vi "Joystick Get.vi"(8 "reset":bool, 9 "JoystickRefDrive 2":T2={"Device"=enum."USB 1"}, 10 "JoystickRefOp":T2={"Device"=enum."USB 1"}, 11 "JoystickRefDrive":T2={"Device"=enum."USB 1"}) -> ()   [LabVIEW 2014]
uses:
  <vilib>/Rock Robotics/WPI/Joystick/WPI_JoystickDevRef.ctl
  <vilib>/Rock Robotics/WPI/Joystick/WPI_JoystickDeviceEnum.ctl
  AxisLayoutOpJoyReg.ctl
  ButtonLayoutOpJoyReg.ctl
  ButtonLayoutDriveJoyReg.ctl
  Events.vi
  <vilib>/ptbypt/NI_PtbyPt.lvlib
panel:
  in  "PID gains 2":T1={"proportional gain (Kc)"=0.030222000000000006, "integral time (Ti, min)"=0.025000000000000015, "derivative time (Td, min)"=0.0} {"derivative time (Td, min)" format="%.3f"; "integral time (Ti, min)" format="%.3f"; "proportional gain (Kc)" format="%.3f"}
  in  "PID gains":T1={"proportional gain (Kc)"=2.0, "integral time (Ti, min)"=0.1, "derivative time (Td, min)"=0.0} {"derivative time (Td, min)" format="%.3f"; "integral time (Ti, min)" format="%.3f"; "proportional gain (Kc)" format="%.3f"}
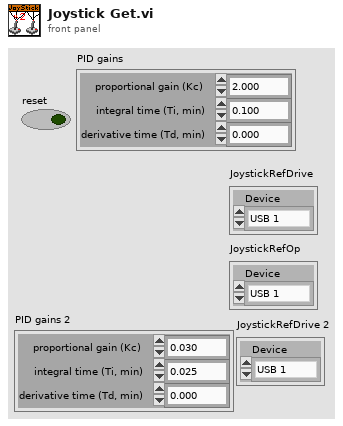
[diagram p1: front panel]
types:
  T1 = cluster{"proportional gain (Kc)":dbl, "integral time (Ti, min)":dbl, "derivative time (Td, min)":dbl}
  T2 = typedef "WPI_JoystickDevRef.ctl" = cluster{"Device":T3}
  T3 = typedef "WPI_JoystickDeviceEnum.ctl" = enum16{"USB 0", "USB 1", "USB 2", "USB 3", "USB 4", "USB 5"}
  T4 = typedef "ButtonLayoutDriveJoyReg.ctl" = cluster{"Ring light":bool, "Button 2":bool, "Button 3":bool, "Button 4":bool, "ShiftLow":bool, "ShiftHigh":bool, "Button 7":bool, "Button 8":bool, " Recalibrate":bool, "Exponential drive":bool, "Button 11":bool, "Button 12":bool}
  T5 = typedef "ButtonLayoutOpJoyReg.ctl" = cluster{"Accq Shoulder":bool, "Reload":bool, "Manuall truss servo":bool, "Button 4":bool, "Pass":bool, "Grab":bool, "Trajectory ctl":bool, "Throw":bool, "Accq Shoulder up":bool, "Button 10":bool, "Button 11":bool, "Button 12":bool}
  T6 = typedef "AxisLayoutOpJoyReg.ctl" = cluster{"axis 1":dbl, "axis 2":dbl, "axis 3":dbl, "axis 4":dbl, "axis 5":dbl, "Change Power":dbl}
  T7 = cluster{"OpJoyType":string, "DriveJoyType":string}
  T8 = cluster{"Translate":dbl, "Y-Axis (Backward Speed)":dbl, "Rotate":dbl, "Tank right side":dbl, "axis 5":dbl, "axis 6":dbl, "Use gyro":bool, "Exponential\ndrive":bool, "Ring light":bool, "PID rotation":bool, "PID Gain":dbl}
  T9 = cluster{"Button 1":bool, "Button 2":bool, "Button 3":bool, "Button 4":bool, "Button 5":bool, "Button 6":bool, "Button 7":bool, "Button 8":bool, "Button 9":bool, "Button 10":bool, "Button 11":bool, "Button 12":bool}
  T10 = cluster{"axis 1 (x)":dbl, "axis 2 (y)":dbl, "axis 3 (throttle)":dbl, "axis 4":dbl, "axis 5":dbl, "axis 6":dbl}
  T11 = typedef "WPI_SolenoidValue.ctl" = enum16{"Off", "On", "Forward", "Reverse"}
  T12 = cluster{"Ultrasonic Distance (In)":dbl, "Gyro":dbl, "TopAquisition sensor":bool, "Encoder distance":dbl, "Encoder rate":dbl, "Encoder direction":bool, "winch engaged?":T11, "Motor Values":dbl[], "Latch encoder":u32, "BottomAquistion":bool, "BottomAquistion 2":bool, "Gyro Rate":dbl}
  T13 = cluster{"axis 1":dbl, "axis 2":dbl, "axis 3":dbl, "axis 4":dbl, "axis 5":dbl, "Change Power":dbl}
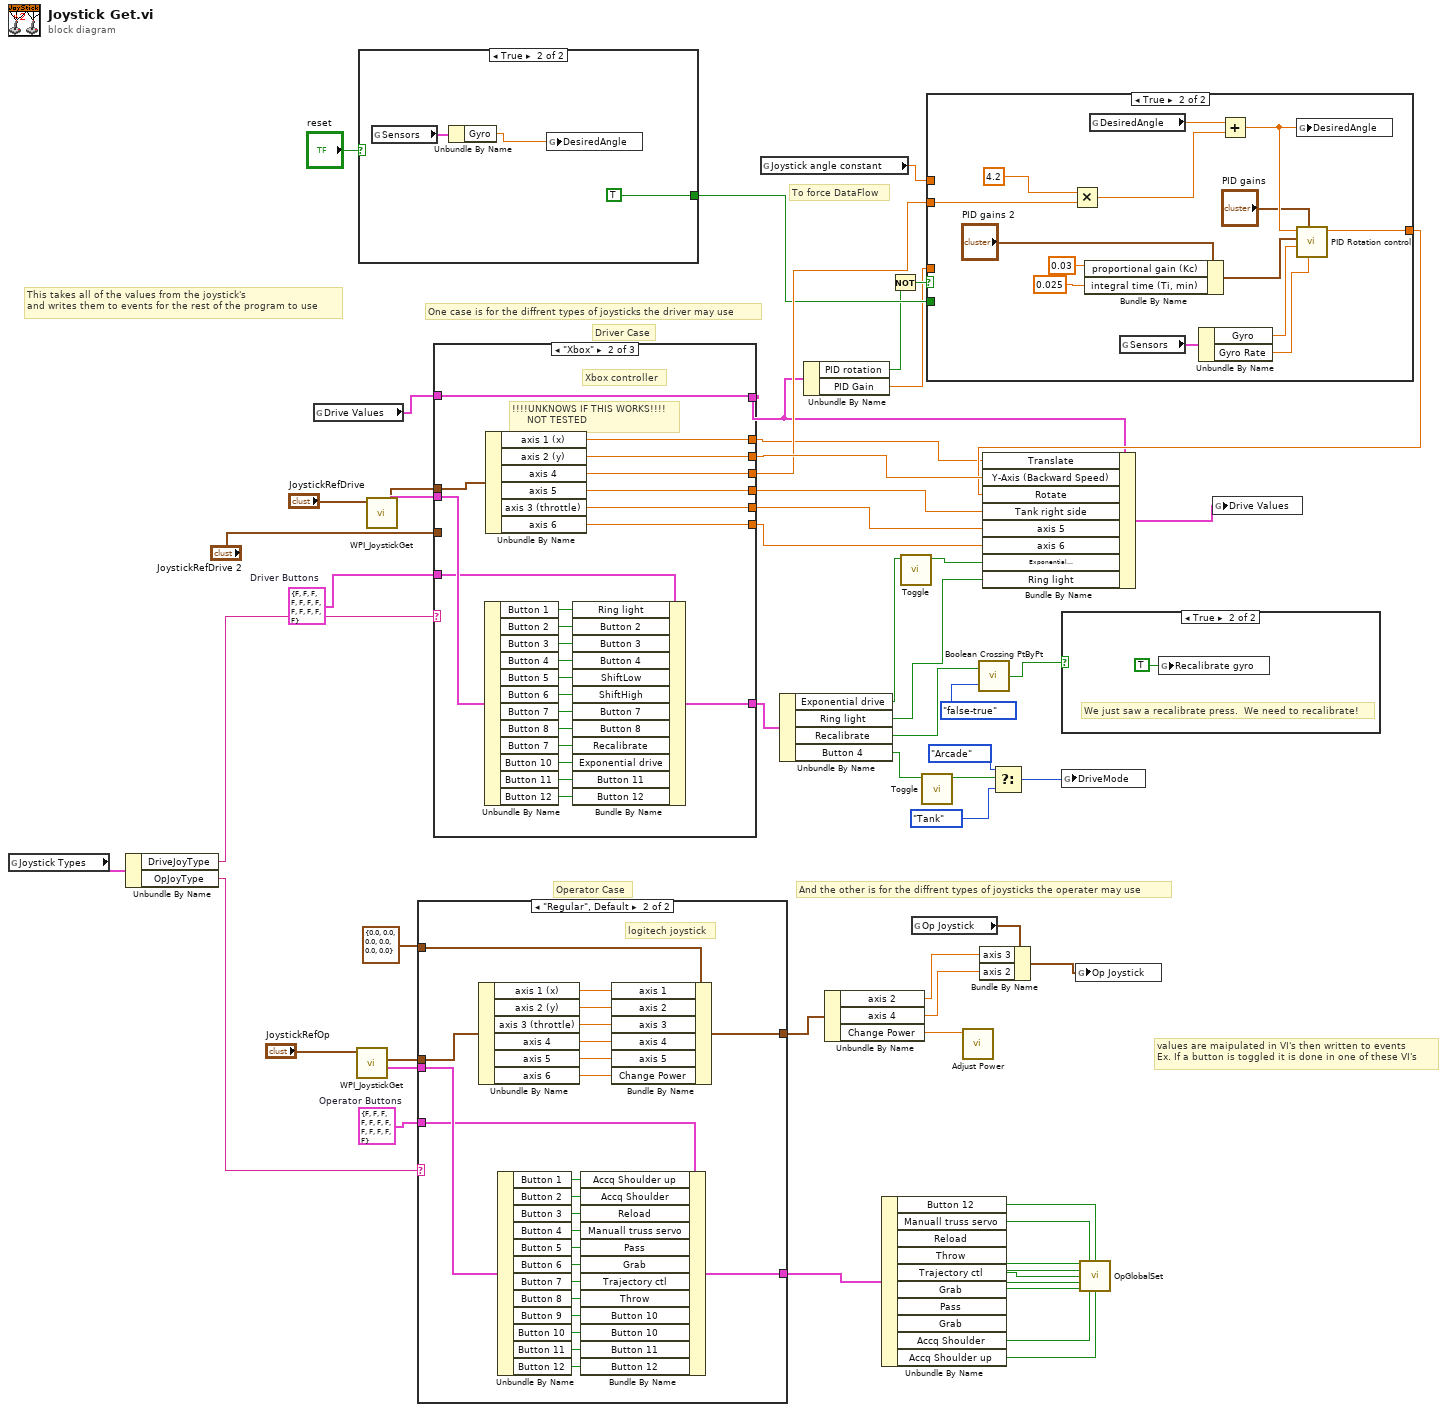
[diagram p0: block diagram]
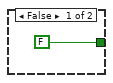
[diagram p2: hidden frame]
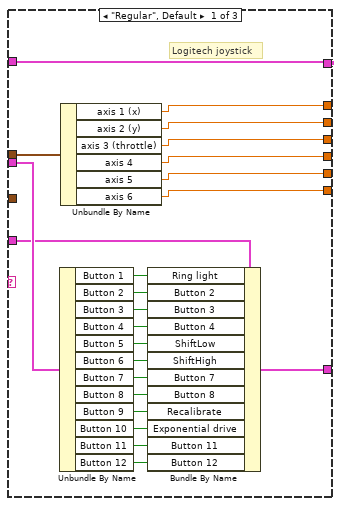
[diagram p5: hidden frame]
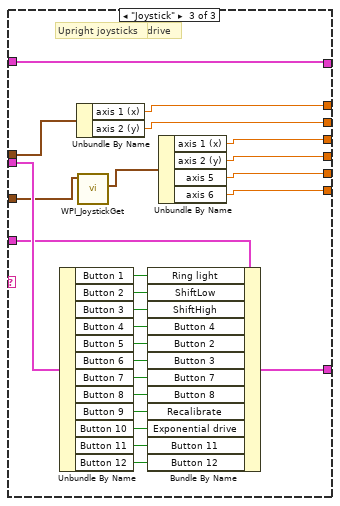
[diagram p6: hidden frame]
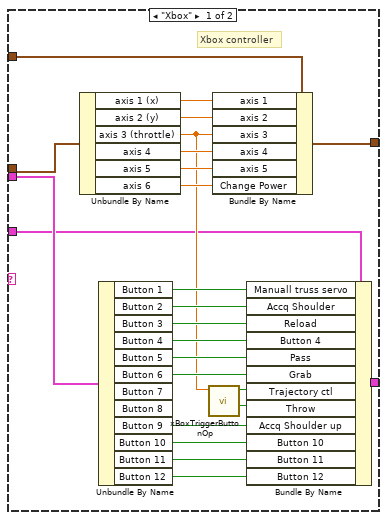
[diagram p7: hidden frame]
diagram:
  w40 = T4 {"Ring light"=FALSE, "Button 2"=FALSE, "Button 3"=FALSE, "Button 4"=FALSE, "ShiftLow"=FALSE, "ShiftHigh"=FALSE, "Button 7"=FALSE, "Button 8"=FALSE, " Recalibrate"=FALSE, "Exponential drive"=FALSE, "Button 11"=FALSE, "Button 12"=FALSE}  # Driver Buttons
  w41 = T5 {"Accq Shoulder"=FALSE, "Reload"=FALSE, "Manuall truss servo"=FALSE, "Button 4"=FALSE, "Pass"=FALSE, "Grab"=FALSE, "Trajectory ctl"=FALSE, "Throw"=FALSE, "Accq Shoulder up"=FALSE, "Button 10"=FALSE, "Button 11"=FALSE, "Button 12"=FALSE}  # Operator Buttons
  # "To force DataFlow"
  # "values are maipulated in VI's then written to events\nEx. If a button is toggled it is done in one of these VI's"
  # "And the other is for the diffrent types of joysticks the operater may use"
  # "One case is for the diffrent types of joysticks the driver may use"
  # "This takes all of the values from the joystick's\nand writes them to events for the rest of the program to use"
  # "Operator Case"
  # "Driver Case"
  n1 = global read "Events.vi" "Joystick Types"() -> (w39:T7)
  n2 = Unbundle By Name(w39) -> ("DriveJoyType"=w18:string, "OpJoyType"=w17:string)
  n3 = global read "Events.vi" "Drive Values"() -> (w38:T8)
  n4 = call <vilib>:"WPI_JoystickGet.vi"("JoystickDevRef"="JoystickRefOp") -> ("Buttons"=w52:T9, "Axes"=w51:T10)  [unwired: 4 in, 1 out]
  n5 = case shown="True" "reset" {
    tunnel: [FALSE TRUE] -> w8
    frame False {
    }
    frame True {
      n6 = global read "Events.vi" "Sensors"() -> (w61:T12)
      n7 = Unbundle By Name(w61) -> ("Gyro"=w59:dbl)
      n8 = global write "Events.vi" "DesiredAngle"(w59) -> ()
    }
  }
  n9 = call <vilib>:"WPI_JoystickGet.vi"("JoystickDevRef"="JoystickRefDrive") -> ("Buttons"=w56:T9, "Axes"=w55:T10)  [unwired: 4 in, 1 out]
  n10 = case shown="\"Regular\", Default" w17 {
    tunnel: w52 -> [w69 w97]
    tunnel: w51 -> [w70 w96]
    tunnel: [w68 w89] -> w50
    tunnel: [w67 w88] -> w43
    tunnel: T6 {"axis 1"=0.0, "axis 2"=0.0, "axis 3"=0.0, "axis 4"=0.0, "axis 5"=0.0, "Change Power"=0.0} ("input cluster") -> [w62 w87]
    tunnel: w41 -> [w63 w86]
    frame "Xbox" {
      # "Xbox controller"
      n11 = Unbundle By Name(w70) -> ("axis 1 (x)"=w75:dbl, "axis 2 (y)"=w74:dbl, "axis 3 (throttle)"=w64:dbl, "axis 4"=w73:dbl, "axis 5"=w72:dbl, "axis 6"=w71:dbl)
      n12 = Unbundle By Name(w69) -> ("Button 1"=w85:bool, "Button 2"=w84:bool, "Button 3"=w83:bool, "Button 4"=w82:bool, "Button 5"=w81:bool, "Button 6"=w80:bool, "Button 9"=w79:bool, "Button 10"=w78:bool, "Button 11"=w77:bool, "Button 12"=w76:bool)  [unwired: 2 out]
      n13 = call "xBoxTriggerButtonOp.vi"("zAxis"=w64) -> ("Throw"=w65:bool, "Lob"=w66:bool)  [unwired: 9 in]
      n14 = Bundle By Name(cluster=w62, "axis 1"=w75, "axis 2"=w74, "axis 3"=w64, "axis 4"=w73, "axis 5"=w72, "Change Power"=w71) -> (w68:T6)
      n15 = Bundle By Name(cluster=w63, "Manuall truss servo"=w85, "Accq Shoulder"=w84, "Reload"=w83, "Button 4"=w82, "Pass"=w81, "Grab"=w80, "Trajectory ctl"=w66, "Throw"=w65, "Accq Shoulder up"=w79, "Button 10"=w78, "Button 11"=w77, "Button 12"=w76) -> (w67:T5)
    }
    frame "Regular", Default {
      # "logitech joystick"
      n16 = Unbundle By Name(w96) -> ("axis 1 (x)"=w95:dbl, "axis 2 (y)"=w94:dbl, "axis 3 (throttle)"=w93:dbl, "axis 4"=w92:dbl, "axis 5"=w91:dbl, "axis 6"=w90:dbl)
      n17 = Unbundle By Name(w97) -> ("Button 1"=w109:bool, "Button 2"=w108:bool, "Button 3"=w107:bool, "Button 4"=w106:bool, "Button 5"=w105:bool, "Button 6"=w104:bool, "Button 7"=w103:bool, "Button 8"=w102:bool, "Button 9"=w101:bool, "Button 10"=w100:bool, "Button 11"=w99:bool, "Button 12"=w98:bool)
      n18 = Bundle By Name(cluster=w86, "Accq Shoulder up"=w109, "Accq Shoulder"=w108, "Reload"=w107, "Manuall truss servo"=w106, "Pass"=w105, "Grab"=w104, "Trajectory ctl"=w103, "Throw"=w102, "Button 10"=w101, "Button 10"=w100, "Button 11"=w99, "Button 12"=w98) -> (w88:T5)
      n19 = Bundle By Name(cluster=w87, "axis 1"=w95, "axis 2"=w94, "axis 3"=w93, "axis 4"=w92, "axis 5"=w91, "Change Power"=w90) -> (w89:T6)
    }
  }
  n20 = case shown="\"Xbox\"" w18 {
    tunnel: w56 -> [w132 w155 w180]
    tunnel: w55 -> [w131 w154 w179]
    tunnel: [w116 w136 w164] -> w7
    tunnel: [w118 w141 w166] -> w54
    tunnel: w38 -> [w116 w136 w164]
    tunnel: w40 -> [w117 w140 w165]
    tunnel: [w115 w139 w163] -> w3
    tunnel: [w114 w138 w162] -> w37
    tunnel: [w113 w133 w161] -> w11
    tunnel: [w112 w134 w160] -> w36
    tunnel: [w111 w135 w159] -> w35
    tunnel: [w110 w137 w158] -> w34
    tunnel: "JoystickRefDrive 2" -> [_ _ w157]
    frame "Regular", Default {
      # "Logitech joystick"
      n21 = Unbundle By Name(w132) -> ("Button 1"=w130:bool, "Button 2"=w129:bool, "Button 3"=w128:bool, "Button 4"=w127:bool, "Button 5"=w126:bool, "Button 6"=w125:bool, "Button 7"=w124:bool, "Button 8"=w123:bool, "Button 9"=w122:bool, "Button 10"=w121:bool, "Button 11"=w120:bool, "Button 12"=w119:bool)
      n22 = Unbundle By Name(w131) -> ("axis 1 (x)"=w115:dbl, "axis 2 (y)"=w114:dbl, "axis 3 (throttle)"=w113:dbl, "axis 4"=w112:dbl, "axis 5"=w111:dbl, "axis 6"=w110:dbl)
      n23 = Bundle By Name(cluster=w117, "Ring light"=w130, "Button 2"=w129, "Button 3"=w128, "Button 4"=w127, "ShiftLow"=w126, "ShiftHigh"=w125, "Button 7"=w124, "Button 8"=w123, "Recalibrate"=w122, "Exponential drive"=w121, "Button 11"=w120, "Button 12"=w119) -> (w118:T4)
    }
    frame "Xbox" {
      # "Xbox controller"
      # "!!!!UNKNOWS IF THIS WORKS!!!!\n     NOT TESTED"
      n24 = Unbundle By Name(w155) -> ("Button 1"=w153:bool, "Button 2"=w152:bool, "Button 3"=w151:bool, "Button 4"=w150:bool, "Button 5"=w149:bool, "Button 6"=w148:bool, "Button 7"=w147:bool, "Button 8"=w146:bool, "Button 7"=w145:bool, "Button 10"=w144:bool, "Button 11"=w143:bool, "Button 12"=w142:bool)
      n25 = Unbundle By Name(w154) -> ("axis 1 (x)"=w139:dbl, "axis 2 (y)"=w138:dbl, "axis 4"=w133:dbl, "axis 5"=w134:dbl, "axis 3 (throttle)"=w135:dbl, "axis 6"=w137:dbl)
      n26 = Bundle By Name(cluster=w140, "Ring light"=w153, "Button 2"=w152, "Button 3"=w151, "Button 4"=w150, "ShiftLow"=w149, "ShiftHigh"=w148, "Button 7"=w147, "Button 8"=w146, "Recalibrate"=w145, "Exponential drive"=w144, "Button 11"=w143, "Button 12"=w142) -> (w141:T4)
    }
    frame "Joystick" {
      # "driver uses two to drive"
      # "Upright joysticks"
      n27 = Unbundle By Name(w180) -> ("Button 1"=w178:bool, "Button 2"=w177:bool, "Button 3"=w176:bool, "Button 4"=w175:bool, "Button 5"=w174:bool, "Button 6"=w173:bool, "Button 7"=w172:bool, "Button 8"=w171:bool, "Button 9"=w170:bool, "Button 10"=w169:bool, "Button 11"=w168:bool, "Button 12"=w167:bool)
      n28 = Unbundle By Name(w179) -> ("axis 1 (x)"=w163:dbl, "axis 2 (y)"=w162:dbl)
      n29 = call <vilib>:"WPI_JoystickGet.vi"("JoystickDevRef"=w157) -> ("Axes"=w156:T10)  [unwired: 4 in, 2 out]
      n30 = Bundle By Name(cluster=w165, "Ring light"=w178, "ShiftLow"=w177, "ShiftHigh"=w176, "Button 4"=w175, "Button 2"=w174, "Button 3"=w173, "Button 7"=w172, "Button 8"=w171, "Recalibrate"=w170, "Exponential drive"=w169, "Button 11"=w168, "Button 12"=w167) -> (w166:T4)
      n31 = Unbundle By Name(w156) -> ("axis 1 (x)"=w161:dbl, "axis 2 (y)"=w160:dbl, "axis 5"=w159:dbl, "axis 6"=w158:dbl)
    }
  }
  n32 = global read "Events.vi" "Joystick angle constant"() -> (w2:dbl)
  n33 = Unbundle By Name(w54) -> ("Exponential drive"=w23:bool, "Ring light"=w20:bool, "Recalibrate"=w33:bool, "Button 4"=w16:bool)
  n34 = Unbundle By Name(w7) -> ("PID rotation"=w6:bool, "PID Gain"=w4:dbl)
  n35 = Unbundle By Name(w50) -> ("axis 2"=w19:dbl, "axis 4"=w25:dbl, "Change Power"=w49:dbl)
  n36 = Unbundle By Name(w43) -> ("Button 12"=w1:bool, "Manuall truss servo"=w22:bool, "Reload"=w48:bool, "Throw"=w47:bool, "Trajectory ctl"=w46:bool, "Grab"=w45:bool, "Pass"=w44:bool, "Accq Shoulder"=w28:bool, "Accq Shoulder up"=w21:bool)  [unwired: 1 out]
  n37 = Not(x=w6) -> (.not. x?=w5:bool)
  n38 = call "Toggle.vi"("input"=w23) -> ("output"=w24:bool)  [unwired: 10 in]
  n39 = global read "Events.vi" "Op Joystick"() -> (w27:T13)
  n40 = call "Toggle.vi"("input"=w16) -> ("output"=w15:bool)  [unwired: 10 in]
  n41 = case shown="True" w5 {
    tunnel: w11 -> [w181 w192]
    tunnel: [w181 w191] -> w10
    tunnel: w8 -> [_ _]
    tunnel: w4 -> [_ _]
    tunnel: w2 -> [_ _]
    frame False {
    }
    frame True {
      n42 = Multiply(x=4.2, y=w192) -> (x*y=w194:dbl)
      n43 = Bundle By Name(cluster="PID gains 2", "proportional gain (Kc)"=0.03, "integral time (Ti, min)"=0.025) -> (w185:T1)
      n44 = global read "Events.vi" "DesiredAngle"() -> (w195:dbl)
      n45 = global read "Events.vi" "Sensors"() -> (w190:T12)
      n46 = Unbundle By Name(w190) -> ("Gyro"=w187:dbl, "Gyro Rate"=w189:dbl)
      n47 = Add(x=w195, y=w194) -> (x+y=w193:dbl)
      n48 = global write "Events.vi" "DesiredAngle"(w193) -> ()
      n49 = call "PID Rotation control.vi"("Gyro Rate"=w189, "PID gains"="PID gains", "Gyro"=w187, "PID gains 2"=w185, "Numeric"=w193) -> ("output"=w191:dbl)  [unwired: 6 in]
    }
  }
  n50 = call "Adjust Power.vi"("D-pad input"=w49) -> ()  [unwired: 11 in]
  n51 = call <vilib>:"Boolean Crossing PtByPt.vi"("direction"=enum16{"either", "false-true", "true-false"}."false-true", "input"=w33) -> ("crossing"=w30:bool)  [unwired: 1 in]
  n52 = Bundle By Name(cluster=w27, "axis 3"=w19, "axis 2"=w25) -> (w26:T13)
  n53 = Bundle By Name(cluster=w7, "Translate"=w3, "Y-Axis (Backward Speed)"=w37, "Rotate"=w10, "Tank right side"=w36, "axis 5"=w35, "axis 6"=w34, "Exponential\ndrive"=w24, "Ring light"=w20) -> (w29:T8)
  n54 = Select(t=enum16{"Arcade", "Tank", "Mecanum"}."Arcade" ("DriveMode"), s=w15, f=enum16{"Arcade", "Tank", "Mecanum"}."Tank" ("DriveMode")) -> (s? t:f=w14:enum16{"Arcade", "Tank", "Mecanum"})
  n55 = case shown="True" w30 {
    frame False {
      # "We don't know that we don't need to recalibrate.\nDon't change anything."
    }
    frame True {
      # "We just saw a recalibrate press.  We need to recalibrate!"
      n56 = global write "Events.vi" "Recalibrate gyro"(TRUE ("Recalibrate gyro")) -> ()
    }
  }
  n57 = global write "Events.vi" "DriveMode"(w14) -> ()
  n58 = global write "Events.vi" "Op Joystick"(w26) -> ()
  n59 = call "OpGlobalSet.vi"("ReloadButton"=w48, "Manuall servo"=w22, "Auton drag"=w1, "ThrowButton"=w47, "LobButton"=w46, "GrabButton"=w45, "GroundPassButton"=w44, "Shoulder joint"=w28, "Shoulder joint up"=w21) -> ()  [unwired: 7 in]
  n60 = global write "Events.vi" "Drive Values"(w29) -> ()
